vi "piezoDoubleWriteDynRegWrite.vi"() -> ()   [LabVIEW 2017]
uses:
  <vilib>/DAQmx/write.llb/DAQmx Write (Analog 2D DBL NChan NSamp).vi
  globalDevices.vi
  globalUtilities.vi
  <vilib>/DAQmx/miscellaneous.llb/DAQmx Fill In Error Info.vi
panel:
  out "success":bool
  out "Waveform Graph 3":dbl[][](graph)
  out "nT":i32
  out "dt":dbl
  out "omega":dbl
  out "amplitude":dbl
  out "offset":dbl
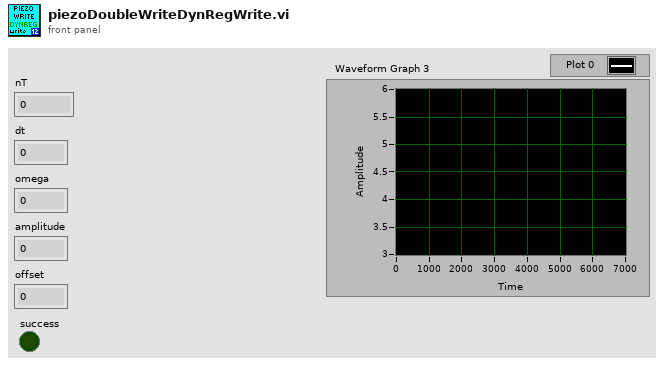
[diagram p1: front panel]
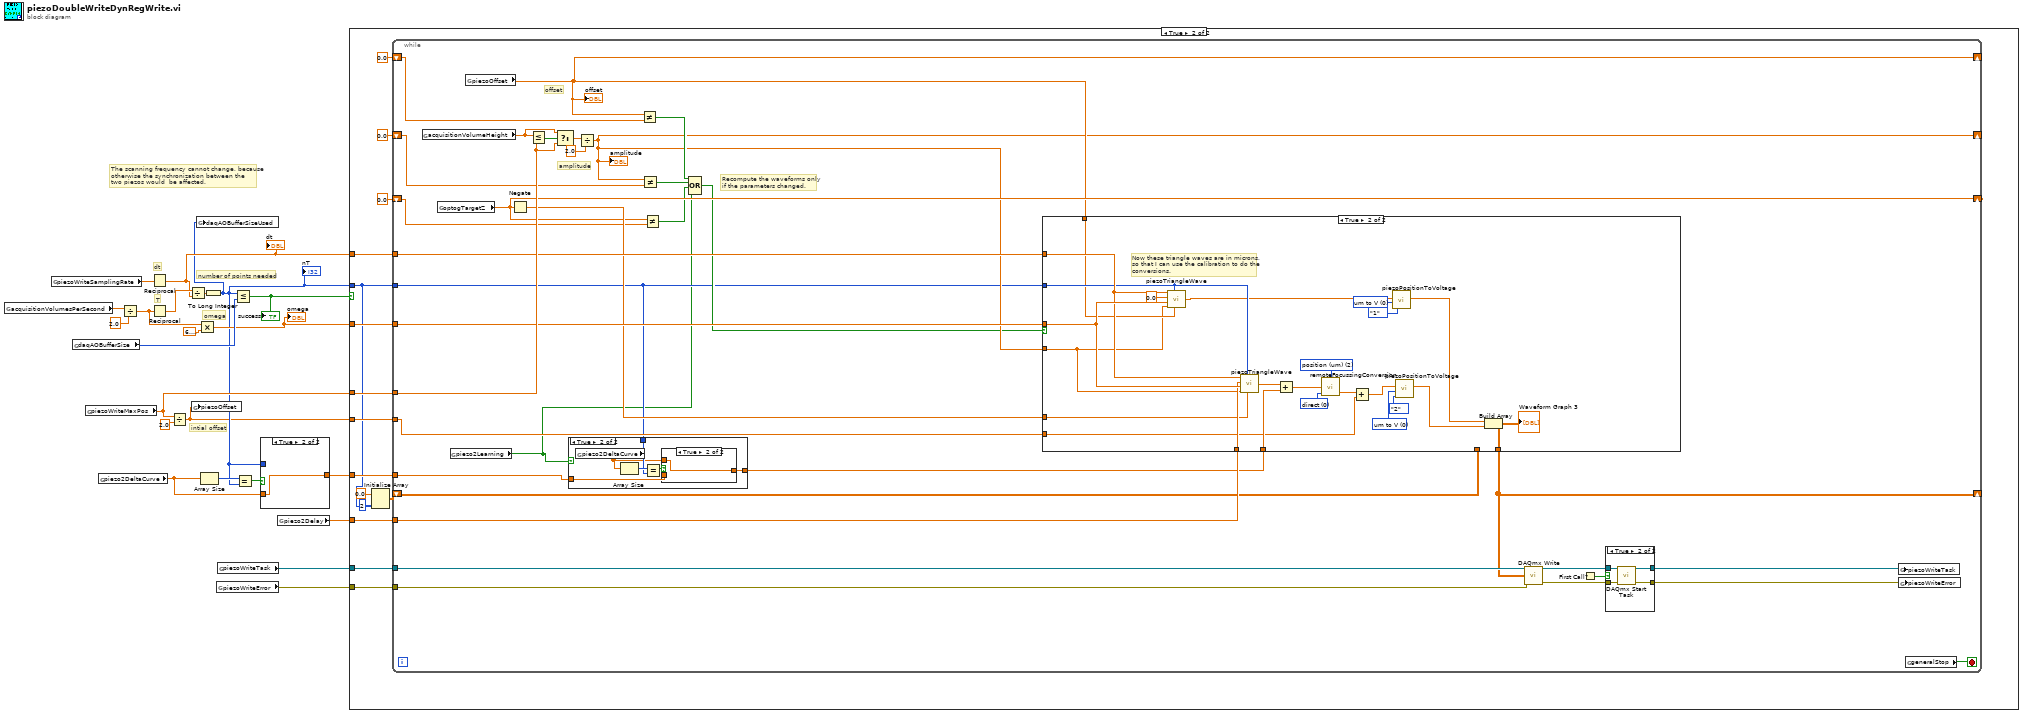
[diagram p0: block diagram]
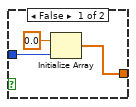
[diagram p7: hidden frame]
diagram:
  # "The scanning frequency cannot change, because\notherwise the synchronization between the \ntwo piezos would  be affected."
  # "omega"
  # "intial offset"
  # "number of points needed"
  # "T"
  # "dt"
  n1 = global read "globalUtilities.vi" "acquisitionVolumesPerSecond"() -> (w19:dbl)
  n2 = global read "globalDevices.vi" "piezoWriteSamplingRate"() -> (w20:dbl)
  n3 = global read "globalDevices.vi" "daqAOBufferSize"() -> (w16:i32)
  n4 = global read "globalDevices.vi" "piezoWriteMaxPos"() -> (w15:dbl)
  n5 = global read "globalDevices.vi" "piezo2DeltaCurve"() -> (w5:dbl[])
  n6 = Divide(x=w19, y=2.0) -> (x/y=w12:dbl)
  n7 = Reciprocal(x=w20) -> (1/x=w10:dbl)
  "dt" <- w10
  n8 = Reciprocal(x=w12) -> (1/x=w17:dbl)
  n9 = Divide(x=w15, y=2.0) -> (x/y=w1:dbl)
  n10 = Divide(x=w17, y=w10) -> (x/y=w8:dbl)
  n11 = global write "globalUtilities.vi" "piezoOffset"(w1) -> ()
  n12 = Multiply(x=w12, y=6.283185307179586) -> (x*y=w11:dbl)
  "omega" <- w11
  n13 = Array Size(array=w5) -> (size(s)=w9:i32)
  n14 = To Long Integer(number=w8) -> (32bit integer=w7:i32)
  "nT" <- w7
  n15 = global write "globalDevices.vi" "daqAOBufferSizeUsed"(w7) -> ()
  n16 = global read "globalDevices.vi" "piezoWriteError"() -> (w22:errorcluster)
  n17 = global read "globalDevices.vi" "piezoWriteTask"() -> (w21:refnum<k21>)
  n18 = Less Or Equal?(x=w7, y=w16) -> (x <= y?=w2:bool)
  "success" <- w2
  n19 = Equal?(x=w9, y=w7) -> (x = y?=w6:bool)
  n20 = case shown="True" w6 {
    tunnel: w7 -> [w24 _]
    tunnel: [w23 w26] -> w4
    tunnel: w5 -> [_ w26]
    frame False {
      n21 = Initialize Array(0.0 ("element"), w24) -> (w23:dbl[])
    }
    frame True {
    }
  }
  n22 = global read "globalDevices.vi" "piezo2Delay"() -> (w3:dbl)
  n23 = case shown="True" w2 {
    tunnel: w22 -> [_ w41]
    tunnel: w21 -> [_ w40]
    tunnel: w15 -> [_ w39]
    tunnel: w11 -> [_ w38]
    tunnel: w10 -> [_ w37]
    tunnel: w7 -> [_ w28]
    tunnel: w4 -> [_ w36]
    tunnel: w3 -> [_ w35]
    tunnel: w1 -> [_ w33]
    frame False {
    }
    frame True {
      n24 = Initialize Array(0.0 ("element"), 2 ("dimension size"), w28) -> (w30:dbl[][])
      n25 = while {
        tunnel: w41 -> [w75]
        tunnel: w40 -> [w74]
        tunnel: w39 -> [w70]
        tunnel: w38 -> [w67]
        tunnel: w37 -> [w66]
        tunnel: w28 -> [w43]
        tunnel: w36 -> [w45]
        tunnel: w35 -> [w64]
        shift-right: [w58] -> _
        shift-left: 0.0 ("targetZ") -> [w59]
        shift-right: [w51] -> _
        shift-left: 0.0 -> [w57]
        shift-right: [w55] -> _
        shift-left: 0.0 ("piezoOffset") -> [w56]
        shift-right: [w50] -> _
        shift-left: w30 -> [w49]
        tunnel: w33 -> [w46]
        stop <- w47 stop-if-true
        # "Recompute the waveforms only\nif the parameters changed."
        # "offset"
        # "amplitude"
        n26 = global read "globalUtilities.vi" "acquisitionVolumeHeight"() -> (w65:dbl)
        n27 = global read "globalUtilities.vi" "optogTargetZ"() -> (w58:dbl)
        n28 = global read "globalDevices.vi" "piezo2Learning"() -> (w42:bool)
        n29 = global read "globalUtilities.vi" "piezoOffset"() -> (w55:dbl)
        "offset" <- w55
        n30 = Negate(x=w58) -> (-x=w60:dbl)
        n31 = Less Or Equal?(x=w65, y=w70) -> (x <= y?=w71:bool)
        n32 = Select(t=w65, s=w71, f=w70) -> (s? t:f=w69:dbl)
        n33 = case shown="True" w42 {
          tunnel: w45 -> [w76 w80]
          tunnel: [w76 w77] -> w44
          tunnel: w43 -> [_ w81]
          frame False {
          }
          frame True {
            n34 = global read "globalDevices.vi" "piezo2DeltaCurve"() -> (w78:dbl[])
            n35 = Array Size(array=w78) -> (size(s)=w82:i32)
            n36 = Equal?(x=w82, y=w81) -> (x = y?=w79:bool)
            n37 = case shown="True" w79 {
              tunnel: w80 -> [w83 _]
              tunnel: w78 -> [_ w84]
              tunnel: [w83 w84] -> w77
              frame False {
              }
              frame True {
              }
            }
          }
        }
        n38 = Divide(x=w69, y=2.0) -> (x/y=w51:dbl)
        "amplitude" <- w51
        n39 = Not Equal?(x=w55, y=w56) -> (x != y?=w54:bool)
        n40 = Not Equal?(x=w51, y=w57) -> (x != y?=w53:bool)
        n41 = Not Equal?(x=w58, y=w59) -> (x != y?=w52:bool)
        n42 = Compound Arithmetic op=OR(w54, w53, w52, w42) -> (w48:bool)
        n43 = case shown="True" w48 {
          tunnel: w67 -> [_ w109]
          tunnel: w66 -> [_ w108]
          tunnel: w43 -> [_ w107]
          tunnel: w44 -> [_ w106]
          tunnel: w64 -> [_ w105]
          tunnel: w60 -> [_ w100]
          tunnel: w55 -> [_ w94]
          tunnel: w51 -> [_ w93]
          tunnel: [w85 w90] -> w50
          tunnel: w49 -> [w85 _]
          tunnel: w46 -> [_ w87]
          frame False {
          }
          frame True {
            w96 = u16 0 items=["um to V", "V to um"] ("mode")
            w99 = u16 0 items=["um to V", "V to um"] ("mode")
            w102 = u16 2 items=["fractional", "voltage (V)", "position (um)"] ("units")
            w103 = u16 0 items=["direct", "inverse"] ("mode")
            # "Now these triangle waves are in microns,\nso that I can use the calibration to do the\nconversions."
            n44 = call "piezoTriangleWave.vi"("offset"=w94, "nT"=w107, "amplitude"=w93, "omega"=w109, "t0"=0.0, "dt"=w108) -> ("x+y"=w97:dbl[])
            n45 = call "piezoTriangleWave.vi"("offset"=w100, "nT"=w107, "amplitude"=w93, "omega"=w109, "t0"=w105, "dt"=w108) -> ("x+y"=w101:dbl[])
            n46 = Add(x=w101, y=w106) -> (x+y=w89:dbl[])
            n47 = call "remoteFocussingConversion.vi"("units"=w102, "mode"=w103, "dz array"=w89) -> ("dz array out"=w88:dbl[])  [unwired: 1 in, 1 out]
            n48 = Add(x=w88, y=w87) -> (x+y=w86:dbl[])
            n49 = call "piezoPositionToVoltage.vi"("piezo"=enum16{"1", "2"}."1", "mode"=w96, "in (array)"=w97) -> ("out (array)"=w92:dbl[])  [unwired: 3 in, 1 out]
            n50 = call "piezoPositionToVoltage.vi"("piezo"=enum16{"1", "2"}."2", "mode"=w99, "in (array)"=w86) -> ("out (array)"=w91:dbl[])  [unwired: 3 in, 1 out]
            n51 = Build Array(w92, w91) -> (w90:dbl[][])
            "Waveform Graph 3" <- w90
          }
        }
        n52 = call-poly <vilib>:"DAQmx Write.vi"("task/channels in"=w74, "data"=w50, "error in"=w75) -> ("task out"=w62:refnum<k21>, "error out"=w63:errorcluster)  [unwired: 10 in, 1 out]
        n53 = First Call?() -> (First Call?: T/F=w61:bool)
        n54 = case shown="True" w61 {
          tunnel: w63 -> [w110 w115]
          tunnel: w62 -> [w111 w114]
          tunnel: [w110 w113] -> w73
          tunnel: [w111 w112] -> w72
          frame False {
          }
          frame True {
            n55 = call <vilib>:"DAQmx Start Task.vi"("task/channels in"=w114, "error in"=w115) -> ("task out"=w112:refnum<k21>, "error out"=w113:errorcluster)  [unwired: 12 in]
          }
        }
        n56 = global write "globalDevices.vi" "piezoWriteTask"(w72) -> ()
        n57 = global write "globalDevices.vi" "piezoWriteError"(w73) -> ()
        n58 = global read "globalUtilities.vi" "generalStop"() -> (w47:bool)
      }
    }
  }
